vi "Load Commiunication Error.vi"(8 "error in (no error)":errorcluster, 11 "main ref":T1) -> (0 "error out":errorcluster)   [LabVIEW 2025]
uses:
  controls/LAB-IQ UI Data.ctl
  <vilib>/Analysis/baseanly.llb/Mean (DBL).vi
  <vilib>/Analysis/NI_AALBase.lvlib
panel:
  out "Load Comflg":bool
  out "OLD VAL":dbl
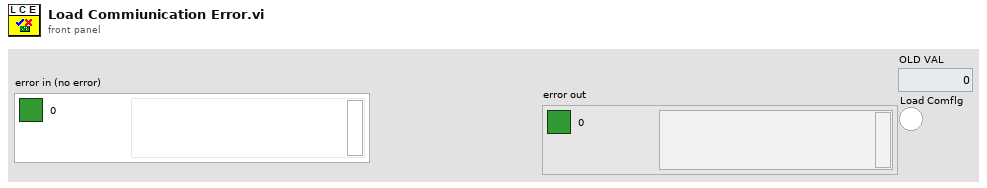
[diagram p1: front panel]
types:
  T1 = typedef "LAB-IQ UI Data.ctl" = cluster{"Main Home Screen":cluster{"GUI":refnum<vi>, "Platform Settings":refnum<vi>, "Configure":refnum<vi>, "Home":refnum<vi>, "EXIT":refnum<vi>, "service 2":refnum<vi>, "MainPage":refnum<vi>, "Analysis":refnum<vi>}, "Platform Settings":cluster{"mm/s  Surge":refnum<vi>, "Update Surge Speed":refnum<vi>, "Drive Error":refnum<vi>, "Disable Axis Jog Soft Limits":refnum<vi>, "mm/s  Sway":refnum<vi>, "Sway and Surge COM Status":refnum<vi>, "Heave COM Status":refnum<vi>, "Enable Platform":refnum<vi>, "Surge Forward Main":refnum<vi>, "Sway Right Main":refnum<vi>, "Sway Left Main":refnum<vi>, "Heave Down Main":refnum<vi>, "Heave Up main":refnum<vi>, "Update Sway Speed":refnum<vi>, "Update Heave Speed":refnum<vi>, "mm/s Heave":refnum<vi>, "mm/sec":refnum<vi>, "mm":refnum<vi>, "Surge Backward Main":refnum<vi>}, "Analysis Screen":cluster{"Analysis Home":refnum<vi>, "Surface Analysis":refnum<vi>, "Imaging":refnum<vi>, "Image Analysis":refnum<vi>, "Post Analysis":refnum<vi>}, "Config Screen":cluster{"Select Load Head":refnum<vi>, "Notes :":refnum<vi>, "FILE":refnum<vi>, "Sample ID :":refnum<vi>, "Operator ID :":refnum<vi>, "Operator Name :":refnum<vi>, "Auto":refnum<vi>}, "Motion Module":cluster{"zNL":refnum<vi>, "NL disp":refnum<vi>, "Rotary Tab":refnum<vi>, "Motion Direction:  3":refnum<vi>, "E.Velocity 2":refnum<vi>, "e.v/ssr 2":refnum<vi>, "Enter Fixed E.Velocity 2":refnum<vi>, "Enter Final SRR 2":refnum<vi>, "Enter initial SRR 2":refnum<vi>, "Enter Fixed SRR 2":refnum<vi>, "Enter the Final E.Velocity (m/s) 2":refnum<vi>, "Enter initial E.Velocity (m/s) 2":refnum<vi>, "Final Speed (RPM) 3":refnum<vi>, "Initial Speed (RPM) 2":refnum<vi>, "Enter the Final Velocity (m/s) 3":refnum<vi>, "Enter initial Velocity (m/s)  3":refnum<vi>, "Ramp Up 2":refnum<vi>, "TEST SELECTION":refnum<vi>, "SPEED SELECTION : ":refnum<vi>, "Angular Oscillation Set":refnum<vi>, "Traction":refnum<vi>, "Step Speed":refnum<vi>, "StepTable For Load-Speed":refnum<vi>, "StepTable For Speed":refnum<vi>, "Surge Forward MM":refnum<vi>, "Surge Backward MM":refnum<vi>, "M3 Image":refnum<vi>, "String 39":refnum<vi>, "Sway Left MM":refnum<vi>, "Sway Right MM":refnum<vi>, "Disable Axis Jog Soft Limits":refnum<vi>, "mm":refnum<vi>, "Heave Down MM":refnum<vi>, "Heave Up MM":refnum<vi>, "Wear Track Diameter (mm)":refnum<vi>, "Set WTD":refnum<vi>, "HomeScratch":refnum<vi>, "HomeRot":refnum<vi>, "PlaceModule":refnum<vi>, "Enter the Angle (Deg)":refnum<vi>, "Enter the Frequency (Hz)":refnum<vi>, "Motion Mode:":refnum<vi>, "LR Sway":refnum<vi>, "Rot Hor":refnum<vi>, "Scratch":refnum<vi>, "LR Cam":refnum<vi>, "MMBack":refnum<vi>, "MMNext":refnum<vi>, "Rot Ver":refnum<vi>, "Rotary Module Selection":refnum<vi>, "calculate rotary":refnum<vi>, "SPEED SELECTION : rotary":refnum<vi>, "Import 2":refnum<vi>, "Save 2":refnum<vi>, "File Path :  2":refnum<vi>, "String 45":refnum<vi>, "StepTable For Speed 3":refnum<vi>, "Enter the Speed(mm/sec)":refnum<vi>, "Enter the Speed(RPM)":refnum<vi>, "Enter Scratch Speed (mm/s):":refnum<vi>, "SwaySpeed Set":refnum<vi>, "Scartch Offset":refnum<vi>, "Motion type:":refnum<vi>, "HomeScratch 2":refnum<vi>, "Enter Scratch length (mm):":refnum<vi>, "Wear Track Diameter":refnum<vi>, "Rotary Speed Exced":refnum<vi>, "Scratch Mode":refnum<vi>, "No of Scratch":refnum<vi>}, "Environmental control":cluster{"Humidity  Status  3":refnum<vi>, "Low Temp  Status  2":refnum<vi>, "TK4 status 2":refnum<vi>, "Stage Temperature":refnum<vi>, "Sample Temperature":refnum<vi>, "Humidity (Amb)":refnum<vi>, "Clear List":refnum<vi>, "Add to list":refnum<vi>, "Wear":refnum<vi>, "Vibration":refnum<vi>, "Humidity (Chamber)":refnum<vi>, "Temperature (Chamber)":refnum<vi>, "ECR ":refnum<vi>, "Temperature (Amb)":refnum<vi>, "Microphone":refnum<vi>, "Acoustic Emission 3":refnum<vi>, "SNext":refnum<vi>, "APBack":refnum<vi>, "Enter the Temperature (°C):":refnum<vi>, "Enter the Stage \nTemperature (°C):":refnum<vi>, "Enter the Humidity (%Rh):":refnum<vi>, "Low Temp":refnum<vi>, "High Temp":refnum<vi>, "Humidity":refnum<vi>, "Sensors Picked":refnum<vi>}, "About Screen":cluster{"Password":refnum<vi>, "Home Service":refnum<vi>, "Advanced Setting":refnum<vi>, "About Tab":refnum<vi>, "ECR Port:":refnum<vi>, "Ramp Port:":refnum<vi>, "Installation/Replacement completed":refnum<vi>, "Loahead":refnum<vi>, "Heave and Surge COM Port:":refnum<vi>, "Sway COM Port:":refnum<vi>, "Temp Modbus:":refnum<vi>, "Humidity Port:":refnum<vi>, "Edit Gain Constants":refnum<vi>, "Save Gain Constants":refnum<vi>}, "Main Screen":cluster{"Main Screen Tab":refnum<vi>, "Angle and Frequency":refnum<vi>, "Stroke (mm)":refnum<vi>, "Angle (Deg)":refnum<vi>, "Main Speed Tab":refnum<vi>, "MTM MOTOR DISPLAY":refnum<vi>, "Disc Speed (m/sec)":refnum<vi>, "Ball Speed (m/sec)":refnum<vi>, "Disc Speed (RPM)":refnum<vi>, "Ball Speed (RPM)":refnum<vi>, "SPEED TAB":refnum<vi>, "Speed (m/sec)":refnum<vi>, "Set Speed (m/sec)":refnum<vi>, "Speed (RPM)":refnum<vi>, "Set Speed":refnum<vi>, "Time Tab":refnum<vi>, "Time ( HH:MM:SS ) 2":refnum<vi>, "Test Duration":refnum<vi>, "Test Duration 4":refnum<vi>, "TEST CYCLE":refnum<vi>, "TOTAL CYCLES":refnum<vi>, "Set Load (N)":refnum<vi>, "Temp Tabs":refnum<vi>, "Heater":refnum<vi>, "TK4 status":refnum<vi>, "ChamberTemp":refnum<vi>, "SetTmp":refnum<vi>, "Controller  Status":refnum<vi>, "ChamberTemp 2":refnum<vi>, "SetTmp 2":refnum<vi>, "Controller  Status 2":refnum<vi>, "ChamberTemp 3":refnum<vi>, "SetTmp 3":refnum<vi>, "Cooling":refnum<vi>, "Load Communication":refnum<vi>, "Ambient \nTemperature":refnum<vi>, "HumCOMStatus":refnum<vi>, "Ambient\n Humidity":refnum<vi>, "Freq (Hz)":refnum<vi>, "Load En":refnum<vi>, "NLt":refnum<vi>, "zNL 2":refnum<vi>, "Humidity On":refnum<vi>, "humidity disp":refnum<vi>, "Set Humidity":refnum<vi>, "NL disp 2":refnum<vi>, "Humidity On 2":refnum<vi>, "humidity disp 2":refnum<vi>, "Set Humidity 2":refnum<vi>, "NL disp 3":refnum<vi>, "AppLoadSeq scratch":refnum<vi>, "Stop Scratch":refnum<vi>, "ClrLog":refnum<vi>, "Trip Log":refnum<vi>, "STOP":refnum<vi>, "Start Test":refnum<vi>, "Test status":refnum<vi>, "AR Led":refnum<vi>, "Data":refnum<vi>, "Health":refnum<vi>, "Sway COM Status":refnum<vi>, "Heave COM Status":refnum<vi>, "Grp Tab":refnum<vi>, "Sub Graph":refnum<vi>, "SD (mm)":refnum<vi>, "Siliding distance Reset Graph":refnum<vi>, "SDGp":refnum<vi>, "Humidity Reset Graph":refnum<vi>, "HumrGp":refnum<vi>, "Acoustic Emission (mV)":refnum<vi>, "Aqucostic Reset Graph":refnum<vi>, "gACQUOS":refnum<vi>, "ECR RESET":refnum<vi>, "ECR":refnum<vi>, "Temperature Reset":refnum<vi>, "Acoustic Emission (mV) 2":refnum<vi>, "Aqucostic Reset Graph 2":refnum<vi>, "gACQUOS 2":refnum<vi>, "ECR RESET 2":refnum<vi>, "ECR 2":refnum<vi>, "Temperature Reset 2":refnum<vi>, "Temperature (deg c)":refnum<vi>, "Speed Reset Graph":refnum<vi>, "Speed Tab":refnum<vi>, "MTM DISC  SPEED":refnum<vi>, "MTM BALL SPEED":refnum<vi>, "speed mm/sec":refnum<vi>, "Hymidity":refnum<vi>, "Humidity Disable trip":refnum<vi>, "CoF Trip  2":refnum<vi>, "Depth Trip":refnum<vi>, "Weart Deapth":refnum<vi>, "Depth Reset Graph":refnum<vi>, "Weart":refnum<vi>, "Depthz":refnum<vi>, "Depth (µm)":refnum<vi>, "WearGp":refnum<vi>, "NL Trip 2":refnum<vi>, "Load pid":refnum<vi>, "Load Disable Trip":refnum<vi>, "Load Reset Graph":refnum<vi>, "NL Display 4":refnum<vi>, "Main Chart 3":refnum<vi>, "BACK":refnum<vi>, "Depth Trip 2":refnum<vi>, "COF TRIP ":refnum<vi>, "Friction Force (N)":refnum<vi>, "FF Reset Graph":refnum<vi>, "FF Disable Trip":refnum<vi>, "FF TRIP":refnum<vi>, "COF Disable Trip":refnum<vi>, "COF Reset Graph":refnum<vi>, "Start Test Temp":refnum<vi>, "zFF":refnum<vi>, "Friction Force (N) Graph":refnum<vi>, "Coefficient of Friction":refnum<vi>, "Scratch Start Test":refnum<vi>, "FF Tab":refnum<vi>, "Cyclic Friction Force (N)":refnum<vi>, "CZ FF":refnum<vi>, "Cyclic Friction Force (N) Graph":refnum<vi>, "Cyclic Coefficient of Friction":refnum<vi>, "Cyclic FF TRIP":refnum<vi>, "Cyclic FF Disable Trip":refnum<vi>, "cyclic COF Disable Trip":refnum<vi>, "cyclic COF TRIP":refnum<vi>, "cyclic COF Reset Graph":refnum<vi>, "Cyclic FF Reset Graph":refnum<vi>, "Test Trip":refnum<vi>, "Multi Scratch Pass":refnum<vi>, "Scratch Start Recording":refnum<vi>}, "Loading":cluster{"Indentation":refnum<vi>, "Reference Sample":refnum<vi>, "Load Cell Communication Slide":refnum<vi>, "com 3":refnum<vi>, "com":refnum<vi>, "DecaForce COM Status":refnum<vi>, "Update":refnum<vi>, "Clear 3":refnum<vi>, "seq":refnum<vi>, "Stribeck table":refnum<vi>, "Stribeck Table  For loading":refnum<vi>, "Loading Mode":refnum<vi>, "Enter the Final Load (N)":refnum<vi>, "Enter the CoF Trip":refnum<vi>, "Enter the Friction Force Trip":refnum<vi>, "Enter the Normal load Trip":refnum<vi>, "Enter the Load  (N)":refnum<vi>, "KiloForce":refnum<vi>, "DecaForce ":refnum<vi>, "MicroForce":refnum<vi>, "LHBack":refnum<vi>, "LHNext":refnum<vi>, "Enter the Loading Rate (N/min)":refnum<vi>, "Message":refnum<vi>, "Warning 2":refnum<vi>, "SSP 0.75":refnum<vi>, "SSP 0.5":refnum<vi>, "SSP 0.3":refnum<vi>, "Warning":refnum<vi>, "gui GIF":refnum<vi>, "Communication is established":refnum<vi>, "AppLoad 4":refnum<vi>, "Multipoint":refnum<vi>, "Load Selection":refnum<vi>}, "PID":cluster{"Ramp MulFac":refnum<vi>, "pulses LoadDiffRamp(2..10)":refnum<vi>, "PulseControlRamp(diff<=3N)":refnum<vi>, "SetLoadDeadband(%) Load(0-10N)":refnum<vi>, "PID gains out delay (microForce)":refnum<vi>, "Ramp":refnum<vi>, "Gain 2":refnum<vi>, "pulses LoadDiff(2..10)":refnum<vi>, "pulses LoadDiff(11..50)":refnum<vi>, "PulseControl(diff<=3N)":refnum<vi>, "SetLoadDeadband(%)  2":refnum<vi>, "Dummy Run":refnum<vi>, "Vertical load (N)":refnum<vi>, "AutoTune":refnum<vi>, "Offset 3 ":refnum<vi>, "apply load":refnum<vi>, "Offset  3":refnum<vi>, "apply load 2":refnum<vi>, "Enter ByPass Load":refnum<vi>, "reinit 3":refnum<vi>, "output range delay":refnum<vi>, "PID gains out delay":refnum<vi>, "Bypass Load":refnum<vi>, "pulsesSent":refnum<vi>, "pulses ":refnum<vi>, "actpid":refnum<vi>, "gFF Rot":refnum<vi>, "pulses LoadDiff(21..1000)":refnum<vi>, "Delay":refnum<vi>, "deadband":refnum<vi>}, "Config Parameters":cluster{"Tab Control 3":refnum<vi>, "Tab Control 19":refnum<vi>, "SAMPLES":refnum<vi>, "Re-initilaize":refnum<vi>, "Filter ON/OFF":refnum<vi>, "TracHomeSurgeOffsetCounts 10MM":refnum<vi>, "TracHomeSwayOffsetCounts 10MM":refnum<vi>, "Acoustic Emission:":refnum<vi>, "Apply Filter (FF)":refnum<vi>, "Filter% 2":refnum<vi>, "Apply Filter (Load)":refnum<vi>, "Filter% ":refnum<vi>, "Sway distance (mm)":refnum<vi>, "Surge distance (mm)":refnum<vi>, "DataSavingLoopDelay(ms)":refnum<vi>, "SAVE 2":refnum<vi>, "Enter Distance":refnum<vi>, "Sway Counts:":refnum<vi>, "Distance (mm): 3":refnum<vi>, "Surge Counts:":refnum<vi>, "Distance (mm): 2":refnum<vi>, "Distance (mm):":refnum<vi>, "Heave Counts:":refnum<vi>, "LRMHomeSurgeOffsetCounts":refnum<vi>, "LRMHomeSwayOffsetCounts":refnum<vi>, "TracHomeSurgeOffsetCounts 20MM":refnum<vi>, "TracHomeSwayOffsetCounts 20MM":refnum<vi>, "RotHomeSwayOffsetCounts":refnum<vi>, "RotHomeSurgeOffsetCounts":refnum<vi>, "Heave distance":refnum<vi>, "Zmm":refnum<vi>, "Heave Pulses/mm":refnum<vi>, "Surge Pulses/mm":refnum<vi>, "Sway Pulses/mm":refnum<vi>, "Heave Pitch":refnum<vi>, "Surge Pitch":refnum<vi>, "Sway Pitch":refnum<vi>, "Heave PPR":refnum<vi>, "Surge PPR":refnum<vi>, "Sway PPR":refnum<vi>, "Tab Control 5":refnum<vi>, "Tab Control 14":refnum<vi>, "Tab Control 26":refnum<vi>, "AE":refnum<vi>, "Heave Loop Delay":refnum<vi>, "Heave PID Speed":refnum<vi>, "Surge Jog Speed":refnum<vi>, "Heave Jog Speed":refnum<vi>, "Sway Loop Delay":refnum<vi>, "Sway PID Speed":refnum<vi>, "Sway Jog Speed":refnum<vi>, "DEPTH TRIP VALUE":refnum<vi>, "LOAD TRIP VALUE":refnum<vi>, "DEPTH TRIP   ENABLE":refnum<vi>, "LOAD TRIP  ENABLE":refnum<vi>, "CYCLIC FF TRIP VALUE":refnum<vi>, "FF TRIP VALUE":refnum<vi>, "CYCLIC CoF TRIP VALUE":refnum<vi>, "COF TRIP VALUE":refnum<vi>, "CYCLIC COF TRIP  ENABLE":refnum<vi>, "CYCLIC FF TRIP  ENABLE":refnum<vi>, "FF TRIP  ENABLE":refnum<vi>, "COF TRIP  ENABLE":refnum<vi>}, "Loading Com Port":cluster{"ClearAll":refnum<vi>, "Mz(Nm)":refnum<vi>, "My(Nm)":refnum<vi>, "Mx(Nm)":refnum<vi>, "Save Dwell":refnum<vi>, "Mx ":refnum<vi>, "My ":refnum<vi>, "Mz":refnum<vi>, "Fx(N)":refnum<vi>, "Fy(N)":refnum<vi>, "Fz(N)":refnum<vi>, "ZeroAll":refnum<vi>, "Acq Delay (ms)":refnum<vi>, "Burst Delay (ms)":refnum<vi>, "model":refnum<vi>, "SN":refnum<vi>, "FFx(N)":refnum<vi>, "Sensor IP":refnum<vi>, "Port":refnum<vi>, "FFy(N)":refnum<vi>, "Load(N)":refnum<vi>, "delete Handle":refnum<vi>, "Create Handle":refnum<vi>, "ft_data":refnum<vi>, "ft_range":refnum<vi>, "ft_data 2":refnum<vi>, "stop 6":refnum<vi>, "running_flag":refnum<vi>, "ft_udp_handle":refnum<vi>, "get-data-return":refnum<vi>, "get-range-return":refnum<vi>, "zero-return":refnum<vi>, "filter-return":refnum<vi>, "initial-return":refnum<vi>, "deleteHandle-result":refnum<vi>, "Load Cell Temp":refnum<vi>}, "Heave AND Surge":cluster{"SURGE POSE":refnum<vi>, "error out Read":refnum<vi>, "HEAVE POSE":refnum<vi>, "State":refnum<vi>, "Homed":refnum<vi>, "Sequence ID":refnum<vi>, "error out Write":refnum<vi>, "faultCode":refnum<vi>, "Ack ID":refnum<vi>, "SPEED":refnum<vi>, "Distance":refnum<vi>, "Mode Command":refnum<vi>, "Heave and Surge Read":refnum<vi>, "Read Heave Temp":refnum<vi>, "Spare 15":refnum<vi>, "Spare 14":refnum<vi>, "Spare 13":refnum<vi>, "Spare 12":refnum<vi>, "Spare 11":refnum<vi>, "Spare 10":refnum<vi>, "Spare 9":refnum<vi>, "Spare 8":refnum<vi>, "Spare 7":refnum<vi>, "Spare 6":refnum<vi>, "Spare 5":refnum<vi>, "Spare 4":refnum<vi>, "Spare 2":refnum<vi>, "Spare 1":refnum<vi>, "Node Id":refnum<vi>, "Spare 3":refnum<vi>, "SPARE 4":refnum<vi>, "SPARE 3":refnum<vi>, "SPARE 2":refnum<vi>, "SPARE 1":refnum<vi>, "fwMajor":refnum<vi>, "fwMinor":refnum<vi>, "Manual Write":refnum<vi>, "Heave and Surge Write":refnum<vi>}, "New PID LOGIC":cluster{"Fine Tune Zone":refnum<vi>, "PID SDelay":refnum<vi>, "Max_pos_limit":refnum<vi>, "Min_pos_limit":refnum<vi>, "i_limit":refnum<vi>, "pct_scale":refnum<vi>, "Deadband":refnum<vi>, "Kd":refnum<vi>, "Ki":refnum<vi>, "Kp":refnum<vi>, "Current Position":refnum<vi>, "Set Load":refnum<vi>, "Current Load":refnum<vi>, "Pulse delta":refnum<vi>, "Init Step":refnum<vi>, "Max Step Linit":refnum<vi>}, "SWAY ":cluster{"fwMajor":refnum<vi>, "Homed":refnum<vi>, "Rotary POSE":refnum<vi>, "State":refnum<vi>, "SWAY POSE":refnum<vi>, "Ack ID":refnum<vi>, "faultCode":refnum<vi>, "Node Id":refnum<vi>, "fwMinor":refnum<vi>, "Spare 6":refnum<vi>, "Spare 5":refnum<vi>, "Spare 4":refnum<vi>, "Spare 3":refnum<vi>, "Spare 2":refnum<vi>, "Spare 1":refnum<vi>, "Spare 7":refnum<vi>, "SPARE  5":refnum<vi>, "error out Write  SWAY ":refnum<vi>, "error out Read SWAY ":refnum<vi>, "Manual Write SWAY ":refnum<vi>, "SWAY WRITE":refnum<vi>, "SPARE  4":refnum<vi>, "SPARE  3":refnum<vi>, "SPARE 2":refnum<vi>, "SPARE 1":refnum<vi>, "Spare 15":refnum<vi>, "Spare 14":refnum<vi>, "Spare 13":refnum<vi>, "Spare 12":refnum<vi>, "Spare 11":refnum<vi>, "Spare 9":refnum<vi>, "Spare 8":refnum<vi>, "SPEED":refnum<vi>, "Distance":refnum<vi>, "Mode Command":refnum<vi>, "Sequence ID":refnum<vi>, "SWAY READ":refnum<vi>, "Spare 10":refnum<vi>, "Read SWAY Temp":refnum<vi>}, "Analysis Screen":cluster{"Analysis Home":refnum<vi>, "Refresh 2":refnum<vi>, "MEAN 4":refnum<vi>, "SD 4":refnum<vi>, "VARIANCE 4":refnum<vi>, "MEAN  3":refnum<vi>, "SD  3":refnum<vi>, "VARIANCE  3":refnum<vi>, "MEAN 2":refnum<vi>, "SD  2":refnum<vi>, "VARIANCE 2":refnum<vi>, "MEAN":refnum<vi>, "SD":refnum<vi>, "VARIANCE":refnum<vi>, "File 4 Discription":refnum<vi>, "OPEN 4":refnum<vi>, "File Name 4":refnum<vi>, "OPEN 3":refnum<vi>, "File 3 Discription":refnum<vi>, "File Name 3":refnum<vi>, "Y-AXIS":refnum<vi>, "X-AXIS":refnum<vi>, "XY Graph":refnum<vi>, "File Name 2":refnum<vi>, "File Name 1":refnum<vi>, "OPEN 2":refnum<vi>, "OPEN 1":refnum<vi>, "File 1 Discription ":refnum<vi>, "File 2 Discription":refnum<vi>, "Export":refnum<vi>, "File Format":refnum<vi>}}
  T2 = enum8{"Enabled", "Disabled", "Disabled and Grayed Out"}
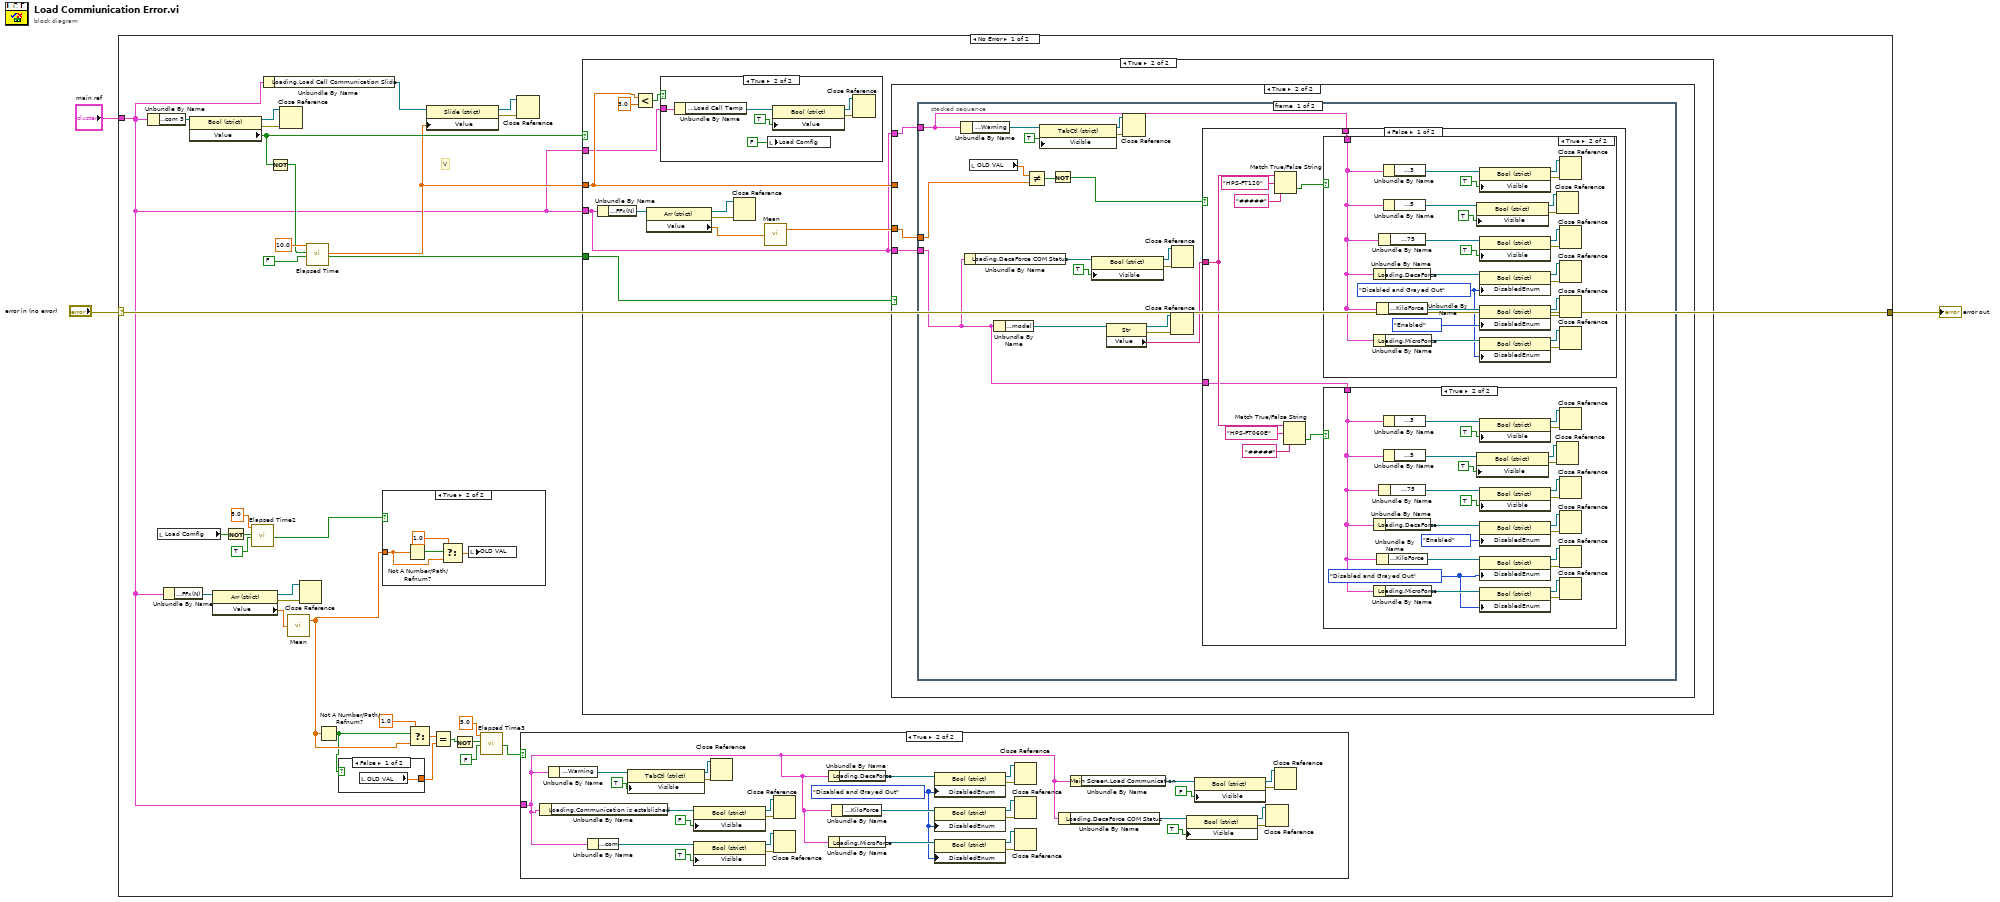
[diagram p0: block diagram]
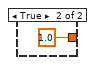
[diagram p2: hidden frame]
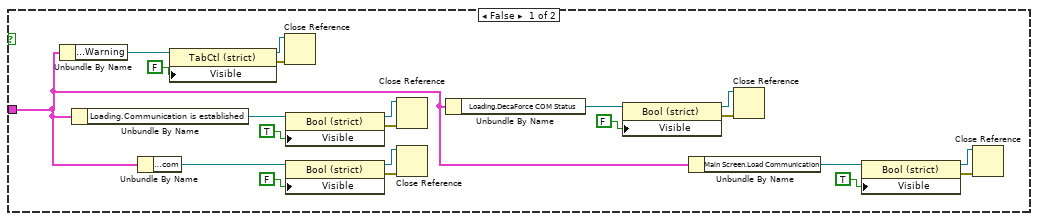
[diagram p3: hidden frame]
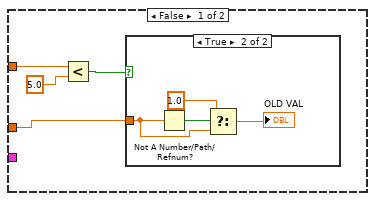
[diagram p7: hidden frame]
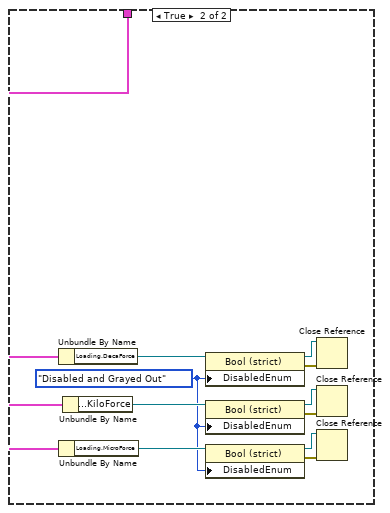
[diagram p11: hidden frame]
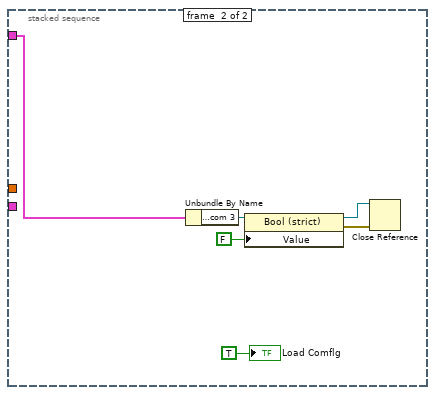
[diagram p12: hidden frame]
diagram:
  n1 = case shown="No Error" "error in (no error)" {
    selector: "error in (no error)" -> [w35 _]
    tunnel: "main ref" -> [w5 _]
    tunnel: [w35 _] -> w1
    frame No Error {
      # "V"
      n2 = Unbundle By Name(w5) -> ("Loading.com 3"=w36:refnum<vi>)
      n3 = local read "Load Comflg"() -> (w23:bool)
      n4 = Unbundle By Name(w5) -> ("Loading Com Port.FFx(N)"=w16:refnum<vi>)
      n5 = property class="Bool (strict)"(reference=w36) -> (reference out=w33:refnum<vi>, error out=w34:errorcluster, "Value"=w31:bool)  [unwired: 1 in]
      n6 = property class="Arr (strict)"(reference=w16) -> (reference out=w18:refnum<vi>, error out=w17:errorcluster, "Value"=w19:dbl[])  [unwired: 1 in]
      n7 = Not(x=w23) -> (.not. x?=w22:bool)
      n8 = call "Elapsed Time2"("Time Target (s)"=5.0, "Reset"=w22, "Auto Reset"=TRUE) -> ("Time has Elapsed"=w15:bool)  [unwired: 9 in, 7 out]
      n9 = Unbundle By Name(w5) -> ("Loading.Load Cell Communication Slide"=w28:refnum<vi>)
      n10 = Not(x=w31) -> (.not. x?=w30:bool)
      n11 = Close Reference(reference=w33, error in (no error)=w34) -> ()  [unwired: 1 out]
      n12 = call-poly <vilib>:"Mean.vi"("X"=w19) -> ("mean"=w13:dbl)  [unwired: 1 out]
      n13 = Close Reference(reference=w18, error in (no error)=w17) -> ()  [unwired: 1 out]
      n14 = call "Elapsed Time"("Time Target (s)"=10.0, "Reset"=w30, "Auto Reset"=FALSE) -> ("Elapsed Time (s)"=w24:dbl, "Time has Elapsed"=w25:bool)  [unwired: 9 in, 6 out]
      n15 = Not A Number/Path/Refnum?(number/path/refnum=w13) -> (NaN/Path/Refnum?=w4:bool)
      n16 = case shown="False" w4 {
        tunnel: [w37 1.0 ("OLD VAL")] -> w11
        frame False {
          n17 = local read "OLD VAL"() -> (w37:dbl)
        }
        frame True {
        }
      }
      n18 = case shown="True" w15 {
        tunnel: w13 -> [_ w92]
        frame False {
        }
        frame True {
          n19 = Not A Number/Path/Refnum?(number/path/refnum=w92) -> (NaN/Path/Refnum?=w94:bool)
          n20 = Select(t=1.0, s=w94, f=w92) -> (s? t:f=w91:dbl)
          n21 = local write "OLD VAL"(w91) -> ()
        }
      }
      n22 = Select(t=1.0, s=w4, f=w13) -> (s? t:f=w12:dbl)
      n23 = property class="Slide (strict)"(reference=w28, "Value"=w24) -> (reference out=w26:refnum<vi>, error out=w27:errorcluster)  [unwired: 1 in]
      n24 = Equal?(x=w12, y=w11) -> (x = y?=w7:bool)
      n25 = Not(x=w7) -> (.not. x?=w8:bool)
      n26 = call "Elapsed Time3"("Time Target (s)"=5.0, "Reset"=w8, "Auto Reset"=FALSE) -> ("Time has Elapsed"=w6:bool)  [unwired: 9 in, 7 out]
      n27 = Close Reference(reference=w26, error in (no error)=w27) -> ()  [unwired: 1 out]
      n28 = case shown="True" w6 {
        tunnel: w5 -> [w39 w60]
        frame False {
          n29 = Unbundle By Name(w39) -> ("Loading.Warning"=w59:refnum<vi>)
          n30 = Unbundle By Name(w39) -> ("Loading.Communication is established"=w53:refnum<vi>)
          n31 = Unbundle By Name(w39) -> ("Loading.com"=w52:refnum<vi>)
          n32 = property class="TabCtl (strict)"(reference=w59, "Visible"=FALSE) -> (reference out=w57:refnum<vi>, error out=w58:errorcluster)  [unwired: 1 in]
          n33 = Close Reference(reference=w57, error in (no error)=w58) -> ()  [unwired: 1 out]
          n34 = property class="Bool (strict)"(reference=w53, "Visible"=TRUE) -> (reference out=w48:refnum<vi>, error out=w54:errorcluster)  [unwired: 1 in]
          n35 = property class="Bool (strict)"(reference=w52, "Visible"=FALSE) -> (reference out=w49:refnum<vi>, error out=w51:errorcluster)  [unwired: 1 in]
          n36 = Close Reference(reference=w48, error in (no error)=w54) -> ()  [unwired: 1 out]
          n37 = Close Reference(reference=w49, error in (no error)=w51) -> ()  [unwired: 1 out]
          n38 = Unbundle By Name(w39) -> ("Loading.DecaForce COM Status"=w47:refnum<vi>)
          n39 = property class="Bool (strict)"(reference=w47, "Visible"=FALSE) -> (reference out=w45:refnum<vi>, error out=w46:errorcluster)  [unwired: 1 in]
          n40 = Unbundle By Name(w39) -> ("Main Screen.Load Communication"=w40:refnum<vi>)
          n41 = Close Reference(reference=w45, error in (no error)=w46) -> ()  [unwired: 1 out]
          n42 = property class="Bool (strict)"(reference=w40, "Visible"=TRUE) -> (reference out=w42:refnum<vi>, error out=w41:errorcluster)  [unwired: 1 in]
          n43 = Close Reference(reference=w42, error in (no error)=w41) -> ()  [unwired: 1 out]
        }
        frame True {
          w70 = T2."Disabled and Grayed Out" ("Disabled")
          n44 = Unbundle By Name(w60) -> ("Loading.Communication is established"=w83:refnum<vi>)
          n45 = Unbundle By Name(w60) -> ("Loading.Warning"=w90:refnum<vi>)
          n46 = Unbundle By Name(w60) -> ("Loading.com"=w82:refnum<vi>)
          n47 = property class="TabCtl (strict)"(reference=w90, "Visible"=TRUE) -> (reference out=w88:refnum<vi>, error out=w89:errorcluster)  [unwired: 1 in]
          n48 = property class="Bool (strict)"(reference=w83, "Visible"=FALSE) -> (reference out=w85:refnum<vi>, error out=w84:errorcluster)  [unwired: 1 in]
          n49 = property class="Bool (strict)"(reference=w82, "Visible"=TRUE) -> (reference out=w69:refnum<vi>, error out=w81:errorcluster)  [unwired: 1 in]
          n50 = Close Reference(reference=w88, error in (no error)=w89) -> ()  [unwired: 1 out]
          n51 = Close Reference(reference=w85, error in (no error)=w84) -> ()  [unwired: 1 out]
          n52 = Close Reference(reference=w69, error in (no error)=w81) -> ()  [unwired: 1 out]
          n53 = Unbundle By Name(w60) -> ("Loading.DecaForce"=w79:refnum<vi>)
          n54 = Unbundle By Name(w60) -> ("Loading.MicroForce"=w74:refnum<vi>)
          n55 = Unbundle By Name(w60) -> ("Loading.KiloForce"=w76:refnum<vi>)
          n56 = property class="Bool (strict)"(reference=w79, "DisabledEnum"=w70) -> (reference out=w71:refnum<vi>, error out=w78:errorcluster)  [unwired: 1 in]
          n57 = property class="Bool (strict)"(reference=w76, "DisabledEnum"=w70) -> (reference out=w75:refnum<vi>, error out=w77:errorcluster)  [unwired: 1 in]
          n58 = property class="Bool (strict)"(reference=w74, "DisabledEnum"=w70) -> (reference out=w72:refnum<vi>, error out=w73:errorcluster)  [unwired: 1 in]
          n59 = Close Reference(reference=w71, error in (no error)=w78) -> ()  [unwired: 1 out]
          n60 = Close Reference(reference=w75, error in (no error)=w77) -> ()  [unwired: 1 out]
          n61 = Close Reference(reference=w72, error in (no error)=w73) -> ()  [unwired: 1 out]
          n62 = Unbundle By Name(w60) -> ("Loading.DecaForce COM Status"=w68:refnum<vi>)
          n63 = Unbundle By Name(w60) -> ("Main Screen.Load Communication"=w62:refnum<vi>)
          n64 = property class="Bool (strict)"(reference=w68, "Visible"=TRUE) -> (reference out=w66:refnum<vi>, error out=w67:errorcluster)  [unwired: 1 in]
          n65 = property class="Bool (strict)"(reference=w62, "Visible"=FALSE) -> (reference out=w64:refnum<vi>, error out=w63:errorcluster)  [unwired: 1 in]
          n66 = Close Reference(reference=w66, error in (no error)=w67) -> ()  [unwired: 1 out]
          n67 = Close Reference(reference=w64, error in (no error)=w63) -> ()  [unwired: 1 out]
        }
      }
      n68 = case shown="True" w31 {
        tunnel: w5 -> [_ w95]
        tunnel: w25 -> [_ w101]
        tunnel: w24 -> [_ w98]
        tunnel: w5 -> [_ w96]
        frame False {
        }
        frame True {
          n69 = Unbundle By Name(w95) -> ("Loading Com Port.FFx(N)"=w105:refnum<vi>)
          n70 = Less?(x=w98, y=3.0) -> (x < y?=w97:bool)
          n71 = property class="Arr (strict)"(reference=w105) -> (reference out=w103:refnum<vi>, error out=w104:errorcluster, "Value"=w102:dbl[])  [unwired: 1 in]
          n72 = case shown="True" w97 {
            tunnel: w96 -> [_ w108]
            frame False {
            }
            frame True {
              n73 = Unbundle By Name(w108) -> ("Loading Com Port.Load Cell Temp"=w111:refnum<vi>)
              n74 = local write "Load Comflg"(FALSE ("Load Comflg")) -> ()
              n75 = property class="Bool (strict)"(reference=w111, "Value"=TRUE) -> (reference out=w109:refnum<vi>, error out=w110:errorcluster)  [unwired: 1 in]
              n76 = Close Reference(reference=w109, error in (no error)=w110) -> ()  [unwired: 1 out]
            }
          }
          n77 = Close Reference(reference=w103, error in (no error)=w104) -> ()  [unwired: 1 out]
          n78 = call-poly <vilib>:"Mean.vi"("X"=w102) -> ("mean"=w100:dbl)  [unwired: 1 out]
          n79 = case shown="True" w101 {
            tunnel: w100 -> [w112 w122]
            tunnel: w98 -> [w115 _]
            tunnel: w95 -> [_ w120]
            tunnel: w95 -> [_ w121]
            frame False {
              n80 = Less?(x=w115, y=5.0) -> (x < y?=w113:bool)
              n81 = case shown="True" w113 {
                tunnel: w112 -> [_ w117]
                frame False {
                }
                frame True {
                  n82 = Not A Number/Path/Refnum?(number/path/refnum=w117) -> (NaN/Path/Refnum?=w119:bool)
                  n83 = Select(t=1.0, s=w119, f=w117) -> (s? t:f=→"OLD VAL":dbl)
                }
              }
            }
            frame True {
              n84 = stacked-sequence {
                tunnel: w122 -> [w139 _]
                tunnel: w121 -> [w124 w212]
                tunnel: w120 -> [w123 _]
                frame #0 {
                  n85 = Unbundle By Name(w124) -> ("Loading.Warning"=w133:refnum<vi>)
                  n86 = Unbundle By Name(w123) -> ("Loading.DecaForce COM Status"=w137:refnum<vi>)
                  n87 = local read "OLD VAL"() -> (w140:dbl)
                  n88 = Unbundle By Name(w123) -> ("Loading Com Port.model"=w126:refnum<vi>)
                  n89 = Not Equal?(x=w140, y=w139) -> (x != y?=w138:bool)
                  n90 = property class="TabCtl (strict)"(reference=w133, "Visible"=TRUE) -> (reference out=w131:refnum<vi>, error out=w132:errorcluster)  [unwired: 1 in]
                  n91 = Not(x=w138) -> (.not. x?=w129:bool)
                  n92 = property class="Bool (strict)"(reference=w137, "Visible"=TRUE) -> (reference out=w135:refnum<vi>, error out=w136:errorcluster)  [unwired: 1 in]
                  n93 = property class="Str"(reference=w126) -> (reference out=w128:refnum<vi>, error out=w127:errorcluster, "Value"=w125:string)  [unwired: 1 in]
                  n94 = Close Reference(reference=w131, error in (no error)=w132) -> ()  [unwired: 1 out]
                  n95 = Close Reference(reference=w128, error in (no error)=w127) -> ()  [unwired: 1 out]
                  n96 = Close Reference(reference=w135, error in (no error)=w136) -> ()  [unwired: 1 out]
                  n97 = case shown="False" w129 {
                    tunnel: w125 -> [w145 _]
                    tunnel: w124 -> [w143 w199]
                    tunnel: w123 -> [w142 _]
                    frame False {
                      n98 = Match True/False String(2:"#####" ("true string"), 3:"HPS-FT120" ("true string"), 4:w145) -> (0:w144:bool)  [unwired: 1 out]
                      n99 = Match True/False String(2:"#####" ("true string"), 3:"HPS-FT060E" ("true string"), 4:w145) -> (0:w141:bool)  [unwired: 1 out]
                      n100 = case shown="True" w144 {
                        tunnel: w143 -> [_ w177]
                        frame False {
                        }
                        frame True {
                          w175 = T2."Disabled and Grayed Out" ("Disabled")
                          n101 = Unbundle By Name(w177) -> ("Loading.DecaForce"=w185:refnum<vi>)
                          n102 = Unbundle By Name(w177) -> ("Loading.MicroForce"=w179:refnum<vi>)
                          n103 = Unbundle By Name(w177) -> ("Loading.KiloForce"=w181:refnum<vi>)
                          n104 = Unbundle By Name(w177) -> ("Loading.SSP 0.75"=w187:refnum<vi>)
                          n105 = Unbundle By Name(w177) -> ("Loading.SSP 0.3"=w195:refnum<vi>)
                          n106 = Unbundle By Name(w177) -> ("Loading.SSP 0.5"=w192:refnum<vi>)
                          n107 = property class="Bool (strict)"(reference=w192, "Visible"=TRUE) -> (reference out=w190:refnum<vi>, error out=w191:errorcluster)  [unwired: 1 in]
                          n108 = property class="Bool (strict)"(reference=w195, "Visible"=TRUE) -> (reference out=w197:refnum<vi>, error out=w196:errorcluster)  [unwired: 1 in]
                          n109 = property class="Bool (strict)"(reference=w187, "Visible"=TRUE) -> (reference out=w189:refnum<vi>, error out=w188:errorcluster)  [unwired: 1 in]
                          n110 = property class="Bool (strict)"(reference=w185, "DisabledEnum"=w175) -> (reference out=w183:refnum<vi>, error out=w184:errorcluster)  [unwired: 1 in]
                          n111 = property class="Bool (strict)"(reference=w181, "DisabledEnum"=T2."Enabled" ("Disabled")) -> (reference out=w180:refnum<vi>, error out=w182:errorcluster)  [unwired: 1 in]
                          n112 = property class="Bool (strict)"(reference=w179, "DisabledEnum"=w175) -> (reference out=w174:refnum<vi>, error out=w178:errorcluster)  [unwired: 1 in]
                          n113 = Close Reference(reference=w190, error in (no error)=w191) -> ()  [unwired: 1 out]
                          n114 = Close Reference(reference=w197, error in (no error)=w196) -> ()  [unwired: 1 out]
                          n115 = Close Reference(reference=w189, error in (no error)=w188) -> ()  [unwired: 1 out]
                          n116 = Close Reference(reference=w183, error in (no error)=w184) -> ()  [unwired: 1 out]
                          n117 = Close Reference(reference=w180, error in (no error)=w182) -> ()  [unwired: 1 out]
                          n118 = Close Reference(reference=w174, error in (no error)=w178) -> ()  [unwired: 1 out]
                        }
                      }
                      n119 = case shown="True" w141 {
                        tunnel: w142 -> [_ w153]
                        frame False {
                        }
                        frame True {
                          w151 = T2."Disabled and Grayed Out" ("Disabled")
                          n120 = Unbundle By Name(w153) -> ("Loading.DecaForce"=w161:refnum<vi>)
                          n121 = Unbundle By Name(w153) -> ("Loading.MicroForce"=w155:refnum<vi>)
                          n122 = Unbundle By Name(w153) -> ("Loading.KiloForce"=w157:refnum<vi>)
                          n123 = Unbundle By Name(w153) -> ("Loading.SSP 0.75"=w163:refnum<vi>)
                          n124 = Unbundle By Name(w153) -> ("Loading.SSP 0.3"=w171:refnum<vi>)
                          n125 = Unbundle By Name(w153) -> ("Loading.SSP 0.5"=w168:refnum<vi>)
                          n126 = property class="Bool (strict)"(reference=w168, "Visible"=TRUE) -> (reference out=w166:refnum<vi>, error out=w167:errorcluster)  [unwired: 1 in]
                          n127 = property class="Bool (strict)"(reference=w171, "Visible"=TRUE) -> (reference out=w173:refnum<vi>, error out=w172:errorcluster)  [unwired: 1 in]
                          n128 = property class="Bool (strict)"(reference=w163, "Visible"=TRUE) -> (reference out=w165:refnum<vi>, error out=w164:errorcluster)  [unwired: 1 in]
                          n129 = property class="Bool (strict)"(reference=w161, "DisabledEnum"=T2."Enabled" ("Disabled")) -> (reference out=w159:refnum<vi>, error out=w160:errorcluster)  [unwired: 1 in]
                          n130 = property class="Bool (strict)"(reference=w157, "DisabledEnum"=w151) -> (reference out=w156:refnum<vi>, error out=w158:errorcluster)  [unwired: 1 in]
                          n131 = property class="Bool (strict)"(reference=w155, "DisabledEnum"=w151) -> (reference out=w152:refnum<vi>, error out=w154:errorcluster)  [unwired: 1 in]
                          n132 = Close Reference(reference=w166, error in (no error)=w167) -> ()  [unwired: 1 out]
                          n133 = Close Reference(reference=w173, error in (no error)=w172) -> ()  [unwired: 1 out]
                          n134 = Close Reference(reference=w165, error in (no error)=w164) -> ()  [unwired: 1 out]
                          n135 = Close Reference(reference=w159, error in (no error)=w160) -> ()  [unwired: 1 out]
                          n136 = Close Reference(reference=w156, error in (no error)=w158) -> ()  [unwired: 1 out]
                          n137 = Close Reference(reference=w152, error in (no error)=w154) -> ()  [unwired: 1 out]
                        }
                      }
                    }
                    frame True {
                      w198 = T2."Disabled and Grayed Out" ("Disabled")
                      n138 = Unbundle By Name(w199) -> ("Loading.DecaForce"=w208:refnum<vi>)
                      n139 = Unbundle By Name(w199) -> ("Loading.MicroForce"=w203:refnum<vi>)
                      n140 = Unbundle By Name(w199) -> ("Loading.KiloForce"=w205:refnum<vi>)
                      n141 = property class="Bool (strict)"(reference=w208, "DisabledEnum"=w198) -> (reference out=w200:refnum<vi>, error out=w207:errorcluster)  [unwired: 1 in]
                      n142 = property class="Bool (strict)"(reference=w205, "DisabledEnum"=w198) -> (reference out=w204:refnum<vi>, error out=w206:errorcluster)  [unwired: 1 in]
                      n143 = property class="Bool (strict)"(reference=w203, "DisabledEnum"=w198) -> (reference out=w201:refnum<vi>, error out=w202:errorcluster)  [unwired: 1 in]
                      n144 = Close Reference(reference=w200, error in (no error)=w207) -> ()  [unwired: 1 out]
                      n145 = Close Reference(reference=w204, error in (no error)=w206) -> ()  [unwired: 1 out]
                      n146 = Close Reference(reference=w201, error in (no error)=w202) -> ()  [unwired: 1 out]
                    }
                  }
                }
                frame #1 {
                  n147 = Unbundle By Name(w212) -> ("Loading.com 3"=w214:refnum<vi>)
                  n148 = property class="Bool (strict)"(reference=w214, "Value"=FALSE) -> (reference out=w211:refnum<vi>, error out=w213:errorcluster)  [unwired: 1 in]
                  n149 = Close Reference(reference=w211, error in (no error)=w213) -> ()  [unwired: 1 out]
                  "Load Comflg" <- TRUE ("Load Comflg")
                }
              }
            }
          }
        }
      }
    }
    frame Error {
    }
  }
  "error out" <- w1
